vi "Save Log File.vi"(0 "file path (use dialog)":path=path "C:/Hitronics_IQC/TestLog/HitronicsTestLog.csv", 7 "VarsIn":T1 {"Pk-Pk" format="%_6f"; "Delay 1-2" format="%_6f"; "Rise" format="%_6f"; "Width" format="%_6f"; "Power Value#2" format="%_6f"; "Power Value#1" format="%_6f"}, 11 "error in":errorcluster) -> (15 "error out":errorcluster)   [LabVIEW 2020]
uses:
  VarsIn.ctl
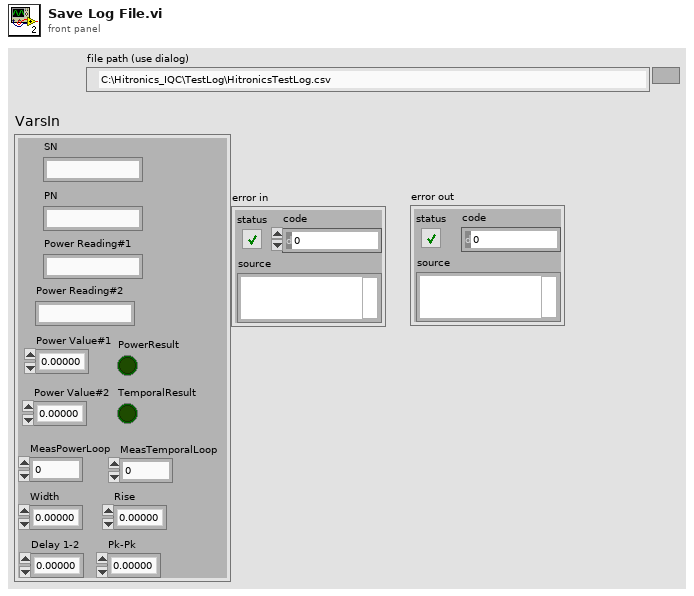
[diagram p1: front panel]
types:
  T1 = typedef "VarsIn.ctl" = cluster{"Power Reading#1":string, "Power Reading#2":string, "SN":string, "PN":string, "Power Value#1":dbl, "Power Value#2":dbl, "MeasPowerLoop":i16, "PowerResult":bool, "Width":dbl, "Rise":dbl, "Delay 1-2":dbl, "Pk-Pk":dbl, "TemporalResult":bool, "MeasTemporalLoop":i16}
  T2 = enum16{"open", "replace", "create", "open or create", "replace or create", "replace or create with confirmation"}
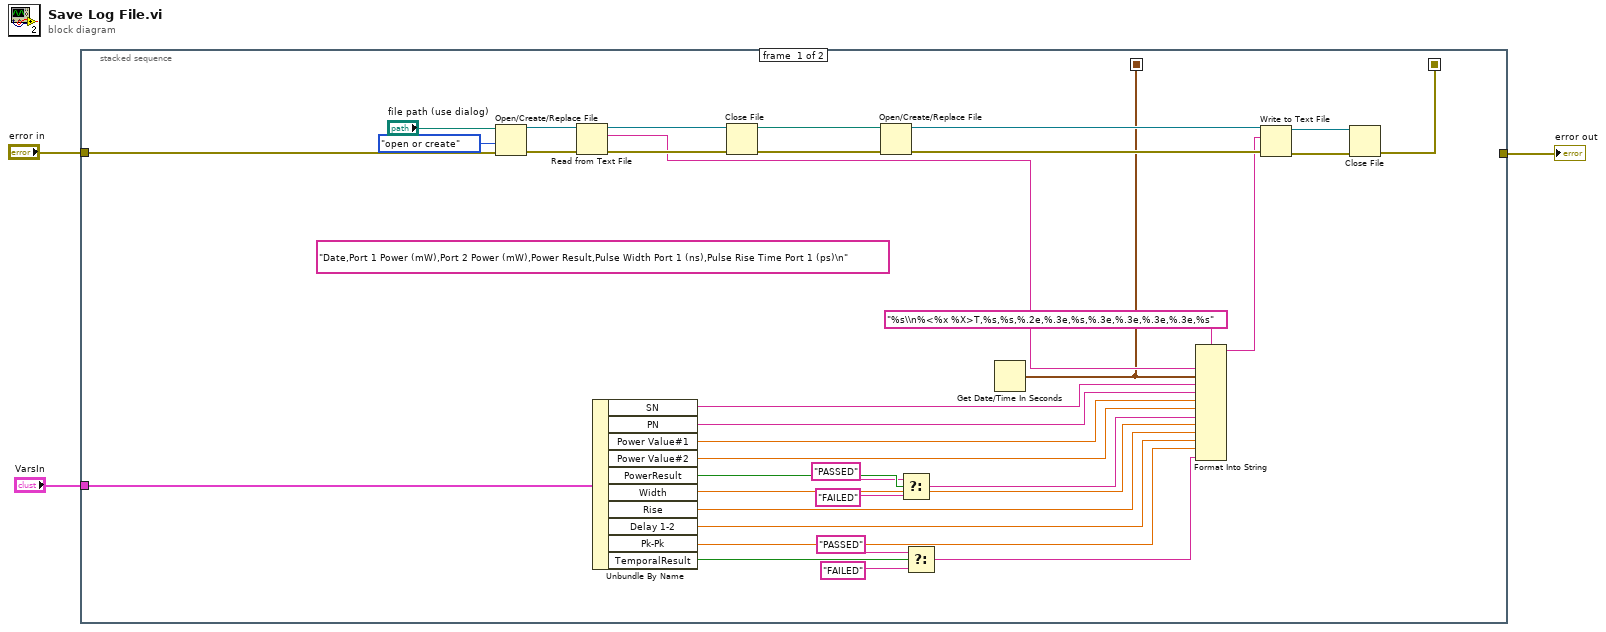
[diagram p0: block diagram]
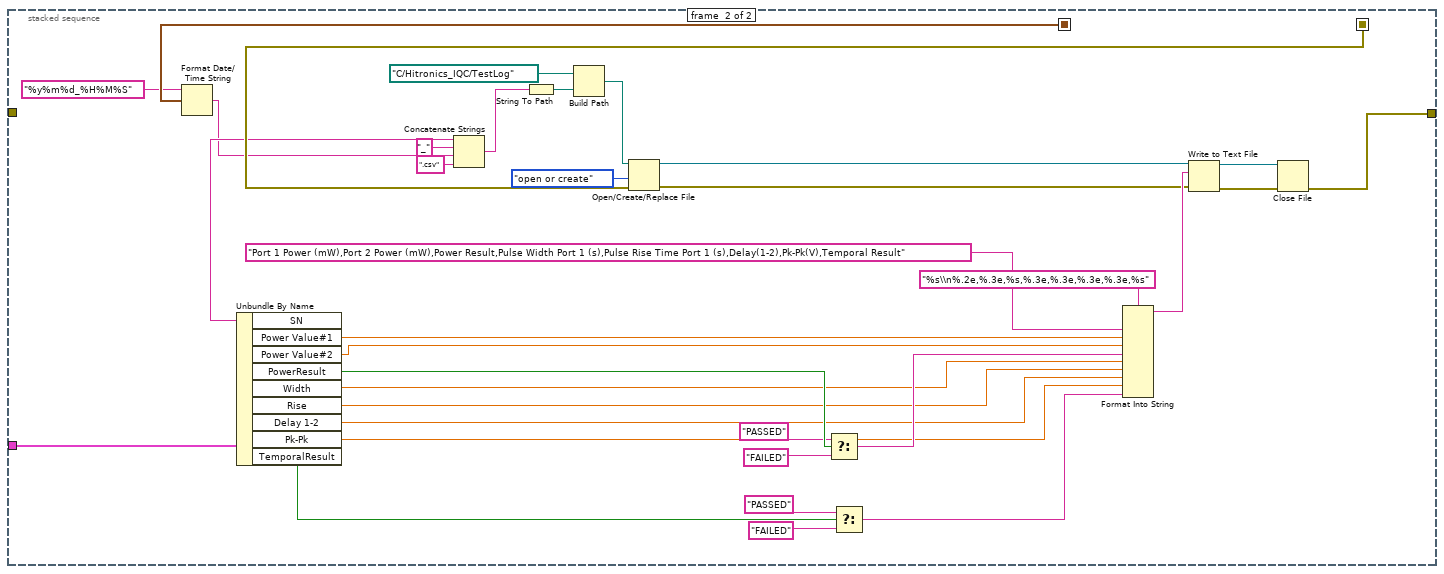
[diagram p2: hidden frame]
diagram:
  n1 = stacked-sequence {
    seq-local: [w5 _] -> [_ w60]
    seq-local: [w4 _] -> [_ w53]
    tunnel: "error in" -> [w7 _]
    tunnel: "VarsIn" -> [w6 w62]
    tunnel: [_ w61] -> w1
    frame #0 {
      (unwired) "Date,Port 1 Power (mW),Port 2 Power (mW),Power Result,Pulse Width Port 1 (ns),Pulse Rise Time Port 1 (ps)\n" ("text")
      n2 = Open/Create/Replace File(file path (use dialog)="file path (use dialog)", error in=w7, operation (0:open)=T2."open or create") -> (refnum out=w33:refnum<file>, error out=w32:errorcluster)  [unwired: 3 in, 1 out]
      n3 = Read from Text File(file (use dialog)=w33, error in=w32) -> (refnum out=w31:refnum<file>, text=w25:string, error out=w30:errorcluster)  [unwired: 2 in, 1 out]
      n4 = Unbundle By Name(w6) -> ("SN"=w23:string, "PN"=w22:string, "Power Value#1"=w21:dbl, "Power Value#2"=w20:dbl, "PowerResult"=w19:bool, "Width"=w12:dbl, "Rise"=w11:dbl, "Delay 1-2"=w10:dbl, "Pk-Pk"=w9:dbl, "TemporalResult"=w13:bool)
      n5 = Close File(refnum=w31, error in=w30) -> (path=w28:path, error out=w27:errorcluster)
      n6 = Open/Create/Replace File(file path (use dialog)=w28, error in=w27) -> (refnum out=w29:refnum<file>, error out=w26:errorcluster)  [unwired: 4 in, 1 out]
      n7 = Select(t="PASSED", s=w19, f="FAILED") -> (s? t:f=w16:string)
      n8 = Select(t="PASSED", s=w13, f="FAILED") -> (s? t:f=w8:string)
      n9 = Get Date/Time In Seconds() -> (seconds since 1Jan1904=w4:timestamp)
      n10 = Format Into String(format string="%s\\n%<%x %X>T,%s,%s,%.2e,%.3e,%s,%.3e,%.3e,%.3e,%.3e,%s", w25, w4, w23, w22, w21, w20, w16, w12, w11, w10, w9, w8) -> (resulting string=w24:string)  [unwired: 2 in, 1 out]
      n11 = Write to Text File(file (use dialog)=w29, text=w24, error in=w26) -> (refnum out=w36:refnum<file>, error out=w35:errorcluster)  [unwired: 1 in, 1 out]
      n12 = Close File(refnum=w36, error in=w35) -> (error out=w5:errorcluster)  [unwired: 1 out]
    }
    frame #1 {
      n13 = Format Date/Time String(time format string (%c)="%y%m%d_%H%M%S", seconds (now)=w53) -> (date/time string=w52:string)  [unwired: 1 in]
      n14 = Unbundle By Name(w62) -> ("SN"=w55:string, "Power Value#1"=w49:dbl, "Power Value#2"=w48:dbl, "PowerResult"=w68:bool, "Width"=w47:dbl, "Rise"=w46:dbl, "Delay 1-2"=w45:dbl, "Pk-Pk"=w44:dbl, "TemporalResult"=w63:bool)
      n15 = Concatenate Strings(w55, "_" ("string"), w52, ".csv" ("string")) -> (w39:string)
      n16 = String To Path(string=w39) -> (path=w42:path)
      n17 = Build Path(base path=path "C:/Hitronics_IQC/TestLog", name or relative path=w42) -> (appended path=w43:path)
      n18 = Open/Create/Replace File(file path (use dialog)=w43, error in=w60, operation (0:open)=T2."open or create") -> (refnum out=w58:refnum<file>, error out=w59:errorcluster)  [unwired: 3 in, 1 out]
      n19 = Select(t="PASSED", s=w68, f="FAILED") -> (s? t:f=w50:string)
      n20 = Select(t="PASSED", s=w63, f="FAILED") -> (s? t:f=w51:string)
      n21 = Format Into String(format string="%s\\n%.2e,%.3e,%s,%.3e,%.3e,%.3e,%.3e,%s", "Port 1 Power (mW),Port 2 Power (mW),Power Result,Pulse Width Port 1 (s),Pulse Rise Time Port 1 (s),Delay(1-2),Pk-Pk(V),Temporal Result" ("text"), w49, w48, w50, w47, w46, w45, w44, w51) -> (resulting string=w69:string)  [unwired: 2 in, 1 out]
      n22 = Write to Text File(file (use dialog)=w58, text=w69, error in=w59) -> (refnum out=w72:refnum<file>, error out=w71:errorcluster)  [unwired: 1 in, 1 out]
      n23 = Close File(refnum=w72, error in=w71) -> (error out=w61:errorcluster)  [unwired: 1 out]
    }
  }
  "error out" <- w1
